vi "FTW-Endpoint-Destroy.vi"(0 "FTW Endpoint":refnum<class "FTW-Endpoint-TCP.lvclass">, 5 "Force Destroy":bool, 11 "error in":errorcluster) -> (15 "error out":errorcluster)   [LabVIEW 2013, in "FTW-Endpoint-TCP.lvclass"]
uses:
  FTW-Endpoint-TCP.lvclass
  FTW-Endpoint-TCP.lvclass/FTW-Endpoint-TCP.ctl
panel:
  # "Inputs"
  # "Outputs"
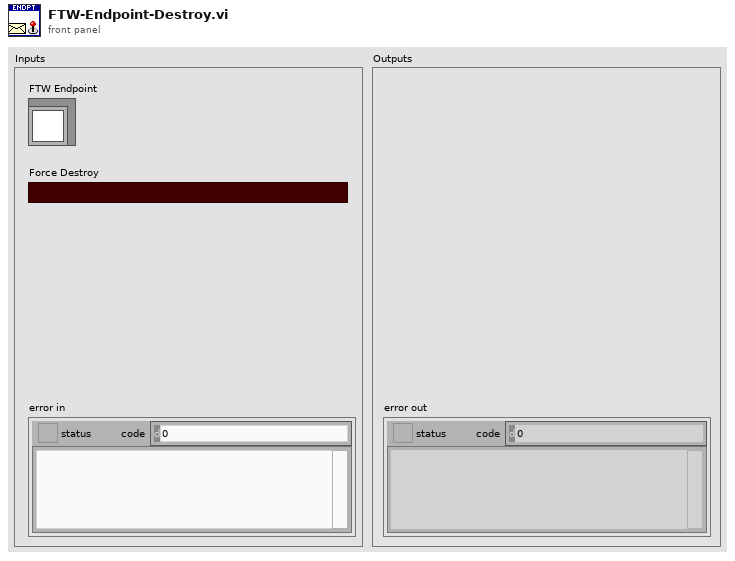
[diagram p1: front panel]
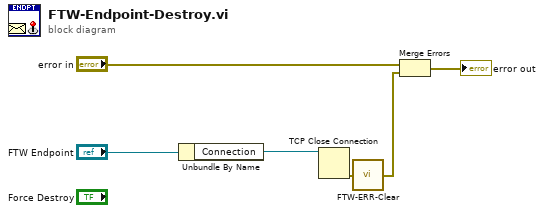
[diagram p0: block diagram]
diagram:
  n1 = Unbundle By Name("FTW Endpoint") -> ("Connection"=w5:refnum<k5>)
  n2 = TCP Close Connection(connection ID=w5) -> (error out=w2:errorcluster)  [unwired: 2 in, 1 out]
  n3 = call "FTW-ERR-Clear.vi"("error to snuff"=w2) -> ("no error"=w1:errorcluster)
  n4 = Merge Errors("error in", w1) -> (→"error out":errorcluster)
